vi "Smart IO Set Pwm Output Period.vi"(8 "error in (no error)":errorcluster, 10 "period":enum16{"20ms", "10ms", "5ms", "2ms"}(ring), 11 "deviceIndex":i32) -> (0 "error out":errorcluster)   [LabVIEW 2026, in "MrcLib.lvlib"]
doc: "Configure the output period of the selected device channel. 20ms is the most compatible option, but you may see operational benefit with faster updates on compatible devices."
uses:
  MrcLib.lvlib
  Types/MRC Smart IO Mode.ctl
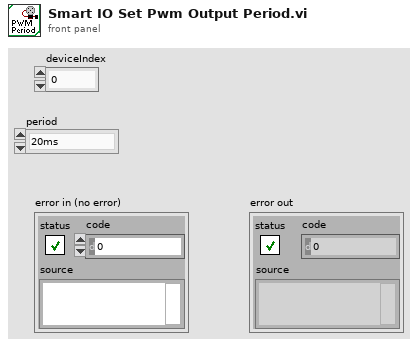
[diagram p1: front panel]
types:
  T1 = typedef "MRC Smart IO Mode.ctl" = i32
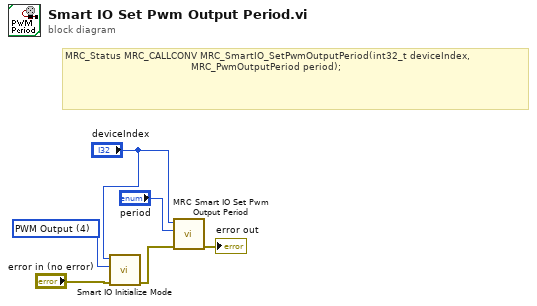
[diagram p0: block diagram]
diagram:
  w1 = T1 4 items=["Digital Input"=0, "Digital Output"=1, "Analog Input"=2, "PWM Input"=3, "PWM Output"=4, "Counter Rising"=5, "Counter Falling"=6, "Addressable LEDs"=13] ("mode")
  # "MRC_Status MRC_CALLCONV MRC_SmartIO_SetPwmOutputPeriod(int32_t deviceIndex,\n                                          MRC_PwmOutputPeriod period);"
  n1 = call "Smart IO Initialize Mode.vi"("error in (no error)"="error in (no error)", "mode"=w1, "deviceIndex"="deviceIndex") -> ("error out"=w4:errorcluster)  [unwired: 8 in]
  n2 = call "MRC Smart IO Set Pwm Output Period.vi"("error in (no error)"=w4, "period"="period", "deviceIndex"="deviceIndex") -> ("error out"=→"error out":errorcluster)  [unwired: 8 in]
